vi "Read PCM channel.vi"(8 "error in (no error)":errorcluster, 11 "Solenoids in":refnum<class "Solenoids.lvclass">) -> (0 "error out":errorcluster, 2 "PCM channel":u8, 3 "Solenoids out":refnum<class "Solenoids.lvclass">)   [LabVIEW 2019, in "Pneumatics control.lvlib" / "Solenoids.lvclass"]
uses:
  Solenoids.lvclass
  Solenoids.lvclass/Solenoids.ctl
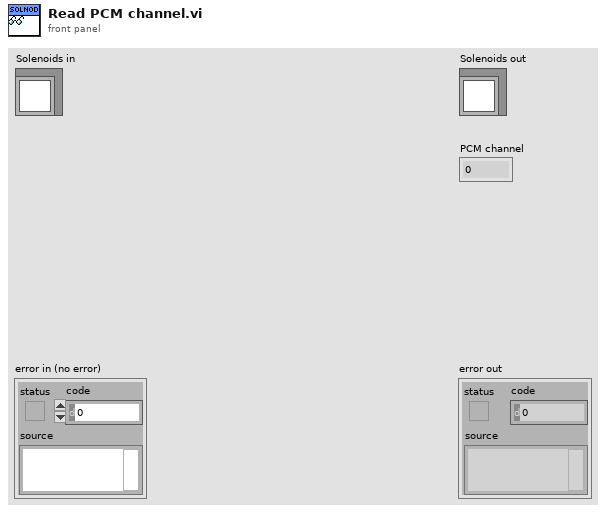
[diagram p1: front panel]
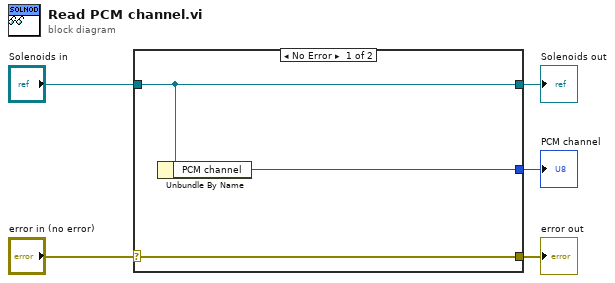
[diagram p0: block diagram]
diagram:
  n1 = case shown="No Error" "error in (no error)" {
    selector: "error in (no error)" -> [w8 w9]
    tunnel: [w8 w9] -> w4
    tunnel: [w7 w10] -> w2
    tunnel: "Solenoids in" -> [w7 w10]
    tunnel: [w6 _] -> w1
    frame No Error {
      n2 = Unbundle By Name(w7) -> ("PCM channel"=w6:u8)
    }
    frame Error {
    }
  }
  "error out" <- w4
  "Solenoids out" <- w2
  "PCM channel" <- w1
